vi "Rio_Theta_Calibration.vi"(8 "error in":errorcluster) -> (0 "error out":errorcluster, 3 "Current Angle Out":i32)   [LabVIEW 2015]
uses:
  <vilib>/myRIO/Common/Instrument Driver Framework/myRIO v1.0/DIO/typedefs/DIO Channels Enum.ctl
  <vilib>/myRIO/Common/Instrument Driver Framework/myRIO v1.0/DIO/typedefs/DIO Channels List.ctl
  <vilib>/myRIO/Common/Instrument Driver Framework/Utilities/typedefs/Generic FPGA Reference.ctl
  <vilib>/myRIO/Common/Instrument Driver Framework/Utilities/typedefs/myRIO v1.0 Reference.ctl
  <vilib>/myRIO/Common/Instrument Driver Framework/Utilities/typedefs/Hardware Version Enum.ctl
  <vilib>/myRIO/Common/Instrument Driver Framework/Utilities/typedefs/myRIO Generic Hardware Reference.ctl
  <vilib>/myRIO/Instrument Drivers/Onboard IO/DIO/typedefs/DIO Reference.ctl
  <vilib>/myRIO/Instrument Drivers/Onboard IO/DIO/DIO.lvlib
  <vilib>/myRIO/Instrument Drivers/Onboard IO/DIO/vis/Write.vi
  <vilib>/userdefined/High Color/nirio_resource_hc.ctl
  <vilib>/myRIO/Common/Instrument Driver Framework/myRIO v1.0/DIO/vis/myRIO v1.1 Open DIO.vi
  <vilib>/myRIO/Instrument Drivers/Onboard IO/DIO/vis/myRIO DIO Open.xnode
  <vilib>/myRIO/Common/Instrument Driver Framework/Utilities/vis/Is FPGA Ref Available.vi
  <vilib>/myRIO/Express VI/Onboard IO/DO/DO Express VI.xnode
  <vilib>/myRIO/Express VI/Onboard IO/DI/DI Express VI.xnode
  <vilib>/myRIO/Instrument Drivers/Onboard IO/DIO/vis/Read.vi
panel:
  out "Theta Limit Switch":bool
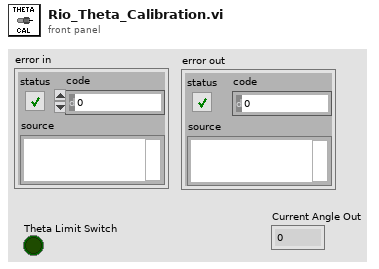
[diagram p1: front panel]
types:
  T1 = typedef "DIO.lvlib/DIO Reference.ctl" = cluster{"myRIO Reference":T2, "DIO Channels List":T6}
  T2 = typedef "myRIO Generic Hardware Reference.ctl" = cluster{"myRIO Model":T3, "myRIO Hardware Reference":T4}
  T3 = typedef "Hardware Version Enum.ctl" = enum16{"Unknown", "myRIO-1900", "myRIO-1950", "roboRIO", "NI ELVIS RIO CM"}
  T4 = typedef "myRIO v1.0 Reference.ctl" = cluster{"Generic FPGA Reference":T5, "Allow multiple opens":bool}
  T5 = typedef "Generic FPGA Reference.ctl" = refnum<k20>
  T6 = typedef "DIO Channels List.ctl" = T7[]
  T7 = typedef "DIO Channels Enum.ctl" = enum16{"Not Connected", "C/DIO0", "C/DIO1", "C/DIO2", "C/DIO3", "C/DIO4", "C/DIO5", "C/DIO6", "C/DIO7", "A/DIO0", "A/DIO1", "A/DIO2", "A/DIO3", "A/DIO4", "A/DIO5", "A/DIO6", "A/DIO7", "A/DIO8", "A/DIO9", "A/DIO10", "A/DIO11", "A/DIO12", "A/DIO13", "A/DIO14", "A/DIO15", "B/DIO0", "B/DIO1", "B/DIO2", "B/DIO3", "B/DIO4", "B/DIO5", "B/DIO6", "B/DIO7", "B/DIO8", "B/DIO9", "B/DIO10", "B/DIO11", "B/DIO12", "B/DIO13", "B/DIO14", "B/DIO15", "LED0", "LED1", "LED2", "LED3", "Button0", "DIO/DIO0", "DIO/DIO1", "DIO/DIO2", "DIO/DIO3", "DIO/DIO4", "DIO/DIO5", "DIO/DIO6", "DIO/DIO7", "DIO/DIO8", "DIO/DIO9", "SPI/CS0", "SPI/CS1", "SPI/CS2", "SPI/CS3", "LED RADIO (Green)", "LED RADIO (Red)", "LED COMM (Green)", "LED COMM (Red)", "LED MODE (Green)", "LED MODE (Red)"}
  T8 = typedef "nirio_resource_hc.ctl" = tag
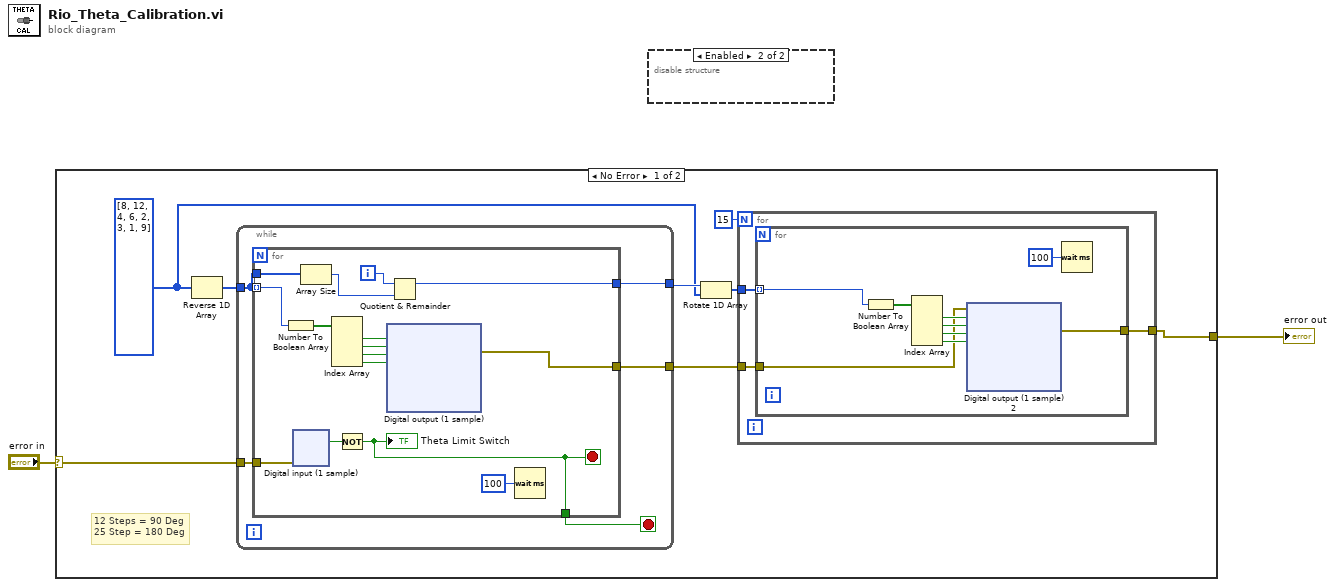
[diagram p0: block diagram]
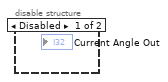
[diagram p2: hidden frame]
diagram:
  n1 = case shown="No Error" "error in" {
    selector: "error in" -> [w9 w154]
    tunnel: [w8 w154] -> w1
    frame No Error {
      w4 = i32[] [8, 12, 4, 6, 2, 3, 1, 9]
      # "12 Steps = 90 Deg\n25 Step = 180 Deg"
      n2 = Reverse 1D Array(array=w4) -> (reversed array=w10:i32[])
      n3 = while {
        tunnel: w10 -> [w62]
        tunnel: [w65] -> w7
        tunnel: w9 -> [w63]
        tunnel: [w61] -> w5
        stop <- w64 stop-if-true
        n4 = for {
          tunnel: w62 -> [w70] mode=indexing
          tunnel: [w74] -> w65
          tunnel: [w72] -> w64
          tunnel: w63 -> [w71]
          tunnel: w62 -> [w68]
          tunnel: [w66] -> w61
          i -> [w69]
          stop <- w72 stop-if-true
          n5 = Number To Boolean Array(number=w70) -> (Boolean array=w80:bool[])
          n6 = xnode ("Digital input (1 sample)")("error in (no error)"=w71) -> ("Theta Limit Switch (A/DIO13 (Pin 26))"=w73:bool)  [unwired: 1 out]
          n7 = Array Size(array=w68) -> (size(s)=w67:i32)
          n8 = Index Array(array=w80) -> (element #1=w79:bool, element #2=w78:bool, element #3=w77:bool, element #4=w76:bool)  [unwired: 4 in]
          n9 = Not(x=w73) -> (.not. x?=w72:bool)
          "Theta Limit Switch" <- w72
          n10 = xnode "Digital output (1 sample)"("0 (A/DIO0 (Pin 11))"=w79, "1 (A/DIO1 (Pin 13))"=w78, "2 (A/DIO2 (Pin 15))"=w77, "3 (A/DIO3 (Pin 17))"=w76) -> ("error out"=w74:errorcluster)  [unwired: 1 in]
          n11 = Quotient & Remainder(x=w69, y=w67) -> (x-y*floor(x/y)=w66:i32)  [unwired: 1 out]
          n12 = Wait (ms)(milliseconds to wait=u32 100) -> ()  [unwired: 1 out]
        }
      }
      n13 = Rotate 1D Array(1:w4, 2:w5) -> (0:w3:i32[])
      n14 = for {
        N: 15 -> [_]
        tunnel: w3 -> [w13]
        tunnel: w7 -> [w11]
        tunnel: [w12] -> w8
        n15 = for {
          tunnel: [w16] -> w12
          tunnel: w13 -> [w15] mode=indexing
          tunnel: w11 -> [w14]
          n16 = Number To Boolean Array(number=w15) -> (Boolean array=w22:bool[])
          n17 = Index Array(array=w22) -> (element #1=w21:bool, element #2=w20:bool, element #3=w19:bool, element #4=w18:bool)  [unwired: 4 in]
          n18 = xnode "Digital output (1 sample) 2"("error in (no error)"=w14, "0 (A/DIO0 (Pin 11))"=w21, "1 (A/DIO1 (Pin 13))"=w20, "2 (A/DIO2 (Pin 15))"=w19, "3 (A/DIO3 (Pin 17))"=w18) -> ("error out"=w16:errorcluster)
          n19 = Wait (ms)(milliseconds to wait=u32 100) -> ()  [unwired: 1 out]
        }
      }
    }
    frame Error {
    }
  }
  "error out" <- w1
  n20 = disable-structure shown="Enabled" {
    frame Disabled {
    }
    frame Enabled {
    }
  }
